vi "test_av_filter.vi"() -> ()   [LabVIEW 2015]
uses:
  <vilib>/sound2/lvsound2.llb/Sound Data Format.ctl
  <vilib>/sound2/lvsound2.llb/Sound File Info (path).vi
  <vilib>/express/express analysis/Spectral/Block/exnSpectralBlock spectral measurements peak poly.vi
  <vilib>/express/express analysis/Spectral/Block/exnSpectralBlock spectral measurements peak array WFM.vi
  <vilib>/express/express analysis/Spectral/XNode/ExpressSpectralMeasurementsBlockNode.xnode
panel:
  in  "path":path
  out "output audio":waveform(dbl)(graph)
  out "sound format":T1={"sample rate (S/s)"=22050.0, "number of channels"=2, "bits per sample"=16}
  out "1/x":dbl
  out "dt":dbl
  out "input audio":waveform(dbl)(graph)
  out "Time-Domain":waveform(dbl)[](graph)
  out "Spectrum":cluster{"f0":dbl, "df":dbl, "magnitude":dbl[]}[](graph)
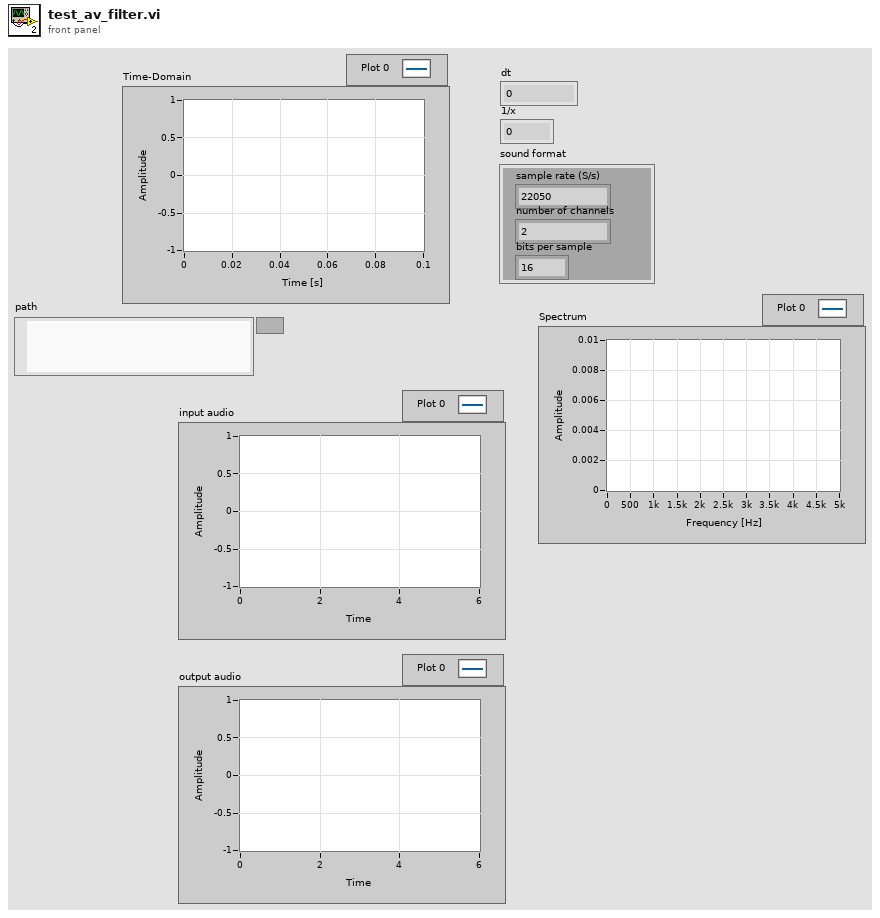
[diagram p1: front panel]
types:
  T1 = typedef "Sound Data Format.ctl" = cluster{"sample rate (S/s)":dbl, "number of channels":i32, "bits per sample":i32}
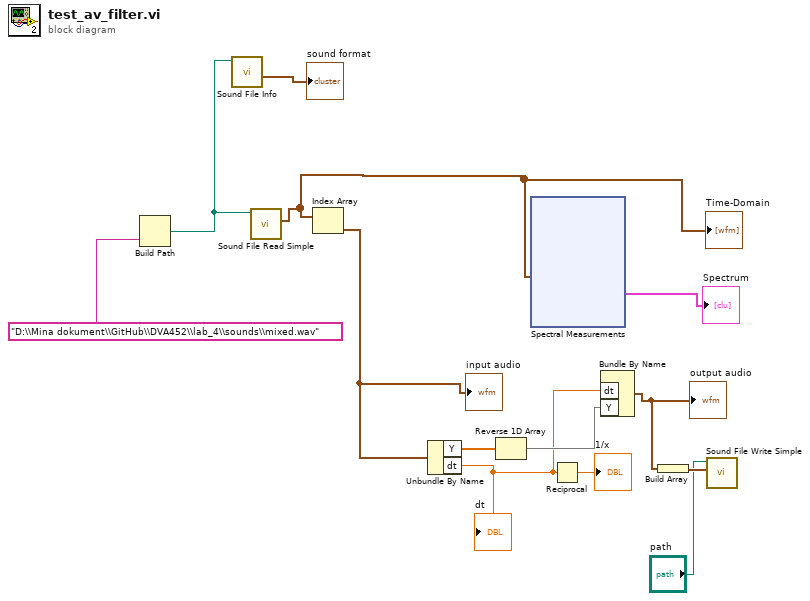
[diagram p0: block diagram]
diagram:
  n1 = Build Path(name or relative path="D:\\Mina dokument\\GitHub\\DVA452\\lab_4\\sounds\\mixed.wav") -> (appended path=w11:path)  [unwired: 1 in]
  n2 = call-poly <vilib>:"Sound File Info.vi"("path"=w11) -> ("sound format"=→"sound format":T1)  [unwired: 7 in, 3 out]
  n3 = call <vilib>:"Sound File Read Simple.vi"("path"=w11) -> ("data"=w1:waveform(dbl)[])  [unwired: 7 in, 3 out]
  "Time-Domain" <- w1
  n4 = Index Array(array=w1) -> (element=w6:waveform(dbl))  [unwired: 1 in]
  "input audio" <- w6
  n5 = Unbundle By Name(w6) -> ("Y"=w12:dbl[], "dt"=w2:dbl)
  "dt" <- w2
  n6 = Reverse 1D Array(array=w12) -> (reversed array=w4:dbl[])
  n7 = xnode "Spectral Measurements"("Signals"=w1) -> ("FFT - (Peak)"=→"Spectrum":cluster{"f0":dbl, "df":dbl, "magnitude":dbl[]}[])  [unwired: 1 in, 2 out]
  n8 = Reciprocal(x=w2) -> (1/x=→"1/x":dbl)
  n9 = Bundle By Name("dt"=w2, "Y"=w4) -> (w5:waveform(dbl))  [unwired: 1 in]
  "output audio" <- w5
  n10 = Build Array(w5) -> (w9:waveform(dbl)[])
  n11 = call <vilib>:"Sound File Write Simple.vi"("data"=w9, "path"="path") -> ()  [unwired: 8 in, 2 out]
